vi "Cov_Light.vi"(11 "Input x":dbl) -> (3 "Light":dbl)   [LabVIEW 2011]
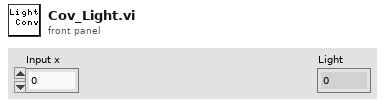
[diagram p1: front panel]
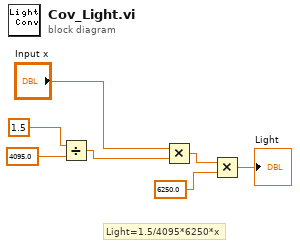
[diagram p0: block diagram]
diagram:
  # "Light=1.5/4095*6250*x"
  n1 = Divide(x=1.5, y=4095.0) -> (x/y=w3:dbl)
  n2 = Multiply(x="Input x", y=w3) -> (x*y=w5:dbl)
  n3 = Multiply(x=w5, y=6250.0) -> (x*y=→"Light":dbl)
